vi "MIDI Controls.vi"(8 "error in (no error)":errorcluster, 10 "MIDI Source":enum16{"Instrument", "File"}(ring)) -> (0 "error out":errorcluster, 3 "MIDI Controls out":variant)   [LabVIEW 2014, in "mySynthesizer.lvlib" / "MIDI Controls.lvlib"]
uses:
  MIDI Controls.lvlib
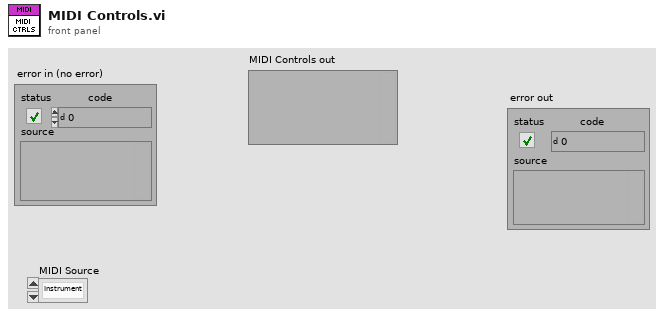
[diagram p1: front panel]
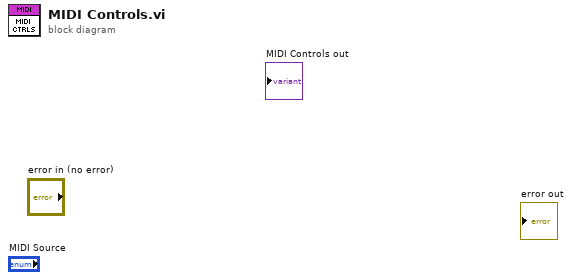
[diagram p0: block diagram]
diagram:
